vi "Error Handler Tester.vi"() -> ()   [LabVIEW 2023]
uses:
  <vilib>/Utility/error.llb/DialogType.ctl
panel:
  in  "Radio Buttons":T1(radio)
  in  "Multiple Errors?":bool
  out "Status Message (Error)":string="Error -2147222150 occurred at Error Handler Tester.vi\r\n\r\nPossible reason(s):\n\nPlease check the specified power sequencing file. The file may be missing, or the power sequence section is not found.\r\n"
  out "error out 3":errorcluster={"status"=TRUE, "code"=56, "source"="Error Handler Tester.vi"}
  in  "error code (0) 4":i32=-2147222150
  in  "error code (0) 3":i32=56
  in  "error code (0) 2":i32=56
  out "message":string="Error -2147222150 occurred at Error Handler Tester.vi\r\n\r\nPossible reason(s):\n\nPlease check the specified power sequencing file. The file may be missing, or the power sequence section is not found."
  out "error out 2":errorcluster={"status"=TRUE, "code"=-2147222150, "source"="Error Handler Tester.vi<ERR>\nPlease check the specified power sequencing file. The file may be missing, or the power sequence section is not found."}
  out "source":string="Error Handler Tester.vi<ERR>\nPlease check the specified power sequencing file. The file may be missing, or the power sequence section is not found."
  in  "error code (0) 1":i32=7
  out "error out":errorcluster={"status"=TRUE, "code"=-2147222150, "source"="Error Handler Tester.vi<ERR>\nPlease check the specified power sequencing file. The file may be missing, or the power sequence section is not found."}
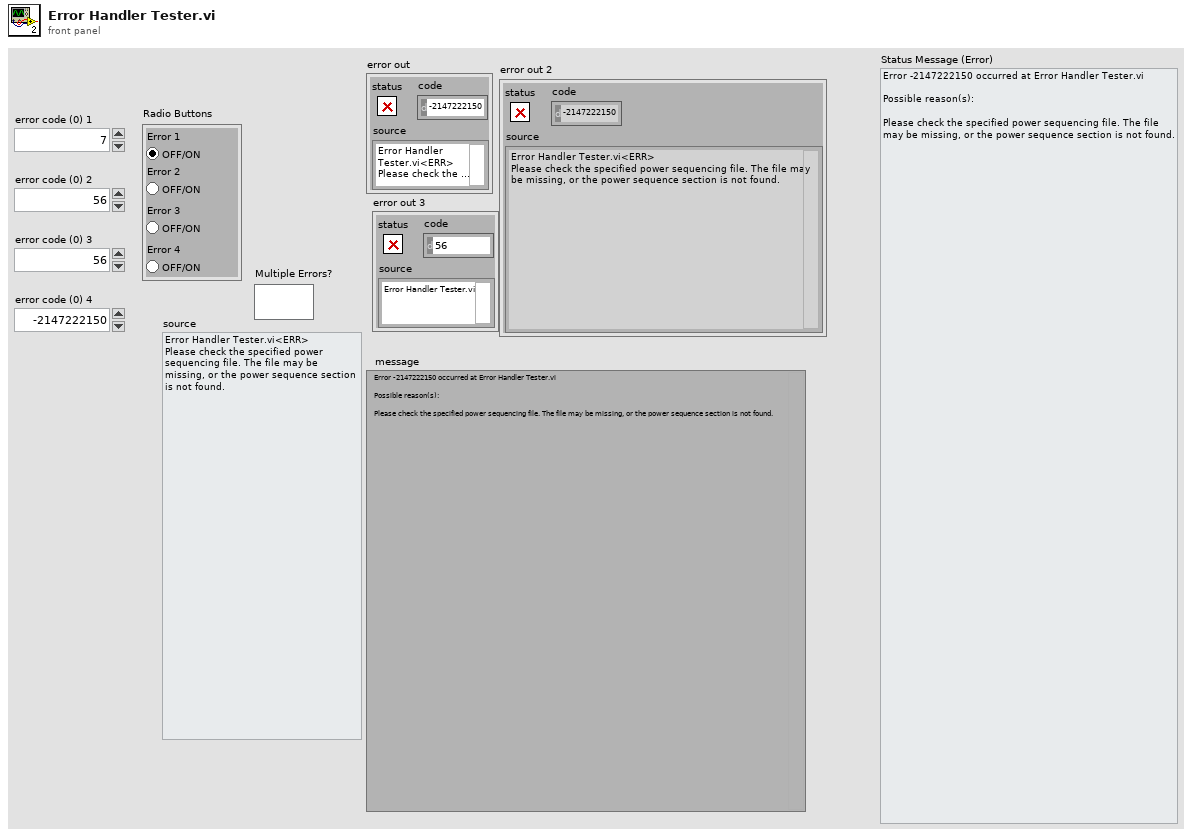
[diagram p1: front panel]
types:
  T1 = enum32{"Error 1", "Error 2", "Error 3", "Error 4"}
  T2 = typedef "DialogType.ctl" = u16
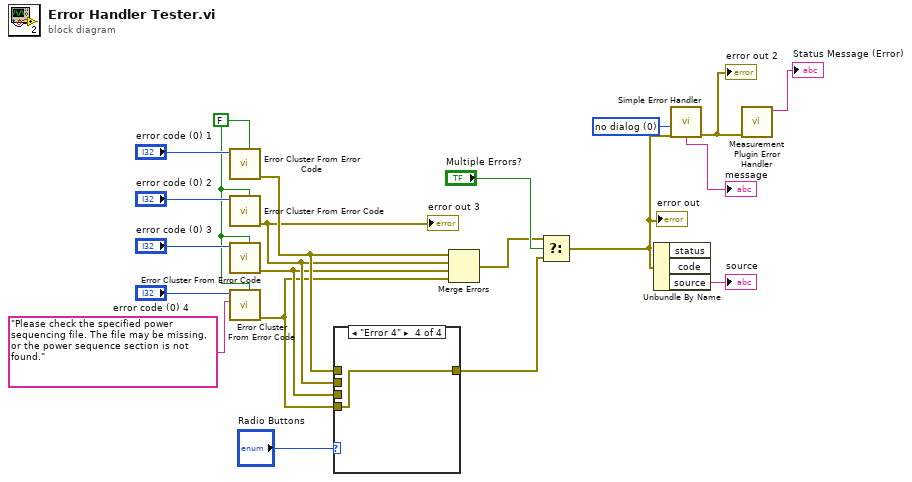
[diagram p0: block diagram]
diagram:
  w10 = FALSE ("is warning? (False)")
  w12 = T2 0 items=["no dialog", "OK message", "continue or stop message", "OK message + warnings", "continue/stop + warnings"] ("type of dialog (OK msg:1)")
  n1 = call <vilib>:"Error Cluster From Error Code.vi"("is warning? (False)"=w10, "error code (0)"="error code (0) 1") -> ("error out"=w5:errorcluster)  [unwired: 7 in]
  n2 = call <vilib>:"Error Cluster From Error Code.vi"("is warning? (False)"=w10, "error code (0)"="error code (0) 2") -> ("error out"=w4:errorcluster)  [unwired: 7 in]
  "error out 3" <- w4
  n3 = call <vilib>:"Error Cluster From Error Code.vi"("is warning? (False)"=w10, "error code (0)"="error code (0) 3") -> ("error out"=w3:errorcluster)  [unwired: 7 in]
  n4 = call <vilib>:"Error Cluster From Error Code.vi"("is warning? (False)"=w10, "error message (\"\")"="Please check the specified power sequencing file. The file may be missing, or the power sequence section is not found." ("error message (\"\")"), "error code (0)"="error code (0) 4") -> ("error out"=w2:errorcluster)  [unwired: 6 in]
  n5 = case shown="\"Error 4\"" "Radio Buttons" {
    tunnel: w5 -> [w21 _ _ _]
    tunnel: w4 -> [_ w22 _ _]
    tunnel: w3 -> [_ _ w23 _]
    tunnel: w2 -> [_ _ _ w24]
    tunnel: [w21 w22 w23 w24] -> w1
    frame "Error 1", Default {
    }
    frame "Error 2" {
    }
    frame "Error 3" {
    }
    frame "Error 4" {
    }
  }
  n6 = Merge Errors(w5, w4, w3, w2) -> (w8:errorcluster)
  n7 = Select(t=w8, s="Multiple Errors?", f=w1) -> (s? t:f=w6:errorcluster)
  "error out" <- w6
  n8 = Unbundle By Name(w6) -> ("source"=→"source":string)  [unwired: 2 out]
  n9 = call <vilib>:"Simple Error Handler.vi"("type of dialog (OK msg:1)"=w12, "error in (no error)"=w6) -> ("error out"=w14:errorcluster, "message"=→"message":string)  [unwired: 3 in, 3 out]
  "error out 2" <- w14
  n10 = call "Measurement Plugin Error Handler.vi"("error in"=w14) -> ("Status Message (Error)"=→"Status Message (Error)":string)  [unwired: 9 in, 1 out]
